vi "p49_1_trinterp.vi"() -> ()   [LabVIEW 2013]
uses:
  <vilib>/robotics/Kinematics/NI_Kinematics.lvlib
panel:
  out "Cartesian Motion 2":refnum<vi>(3d-picture)
  out "size(s) of P":i32[](array[numeric])
  out "Cartesian Motion":refnum<vi>(3d-picture)
  out "Cartesian Position":dbl[][](graph)
  out "RPY":dbl[][](graph)
  out "RPY":dbl[][](graph)
  out "Cartesian Position":dbl[][](graph)
  out "Ts(0)":picture
  out "size(s)":i32[](array[numeric])
  out "transformation matrix":picture
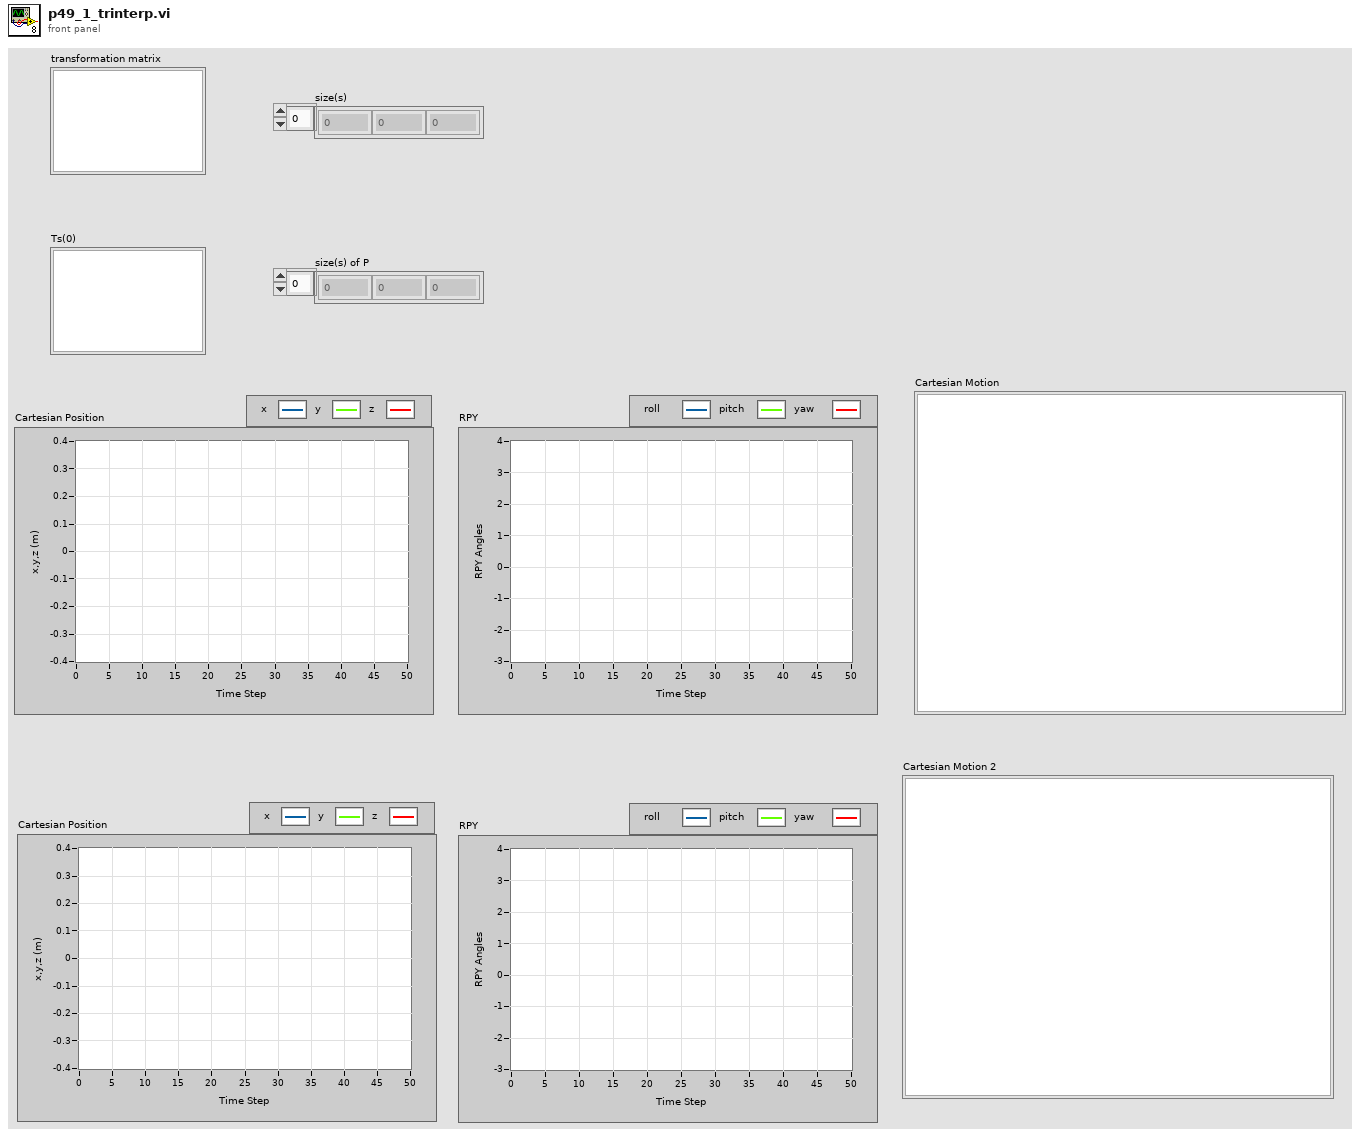
[diagram p1: front panel]
types:
  T1 = typedef "NI_Matrix.lvlib/RealMatrix.ctl" = dbl[][]
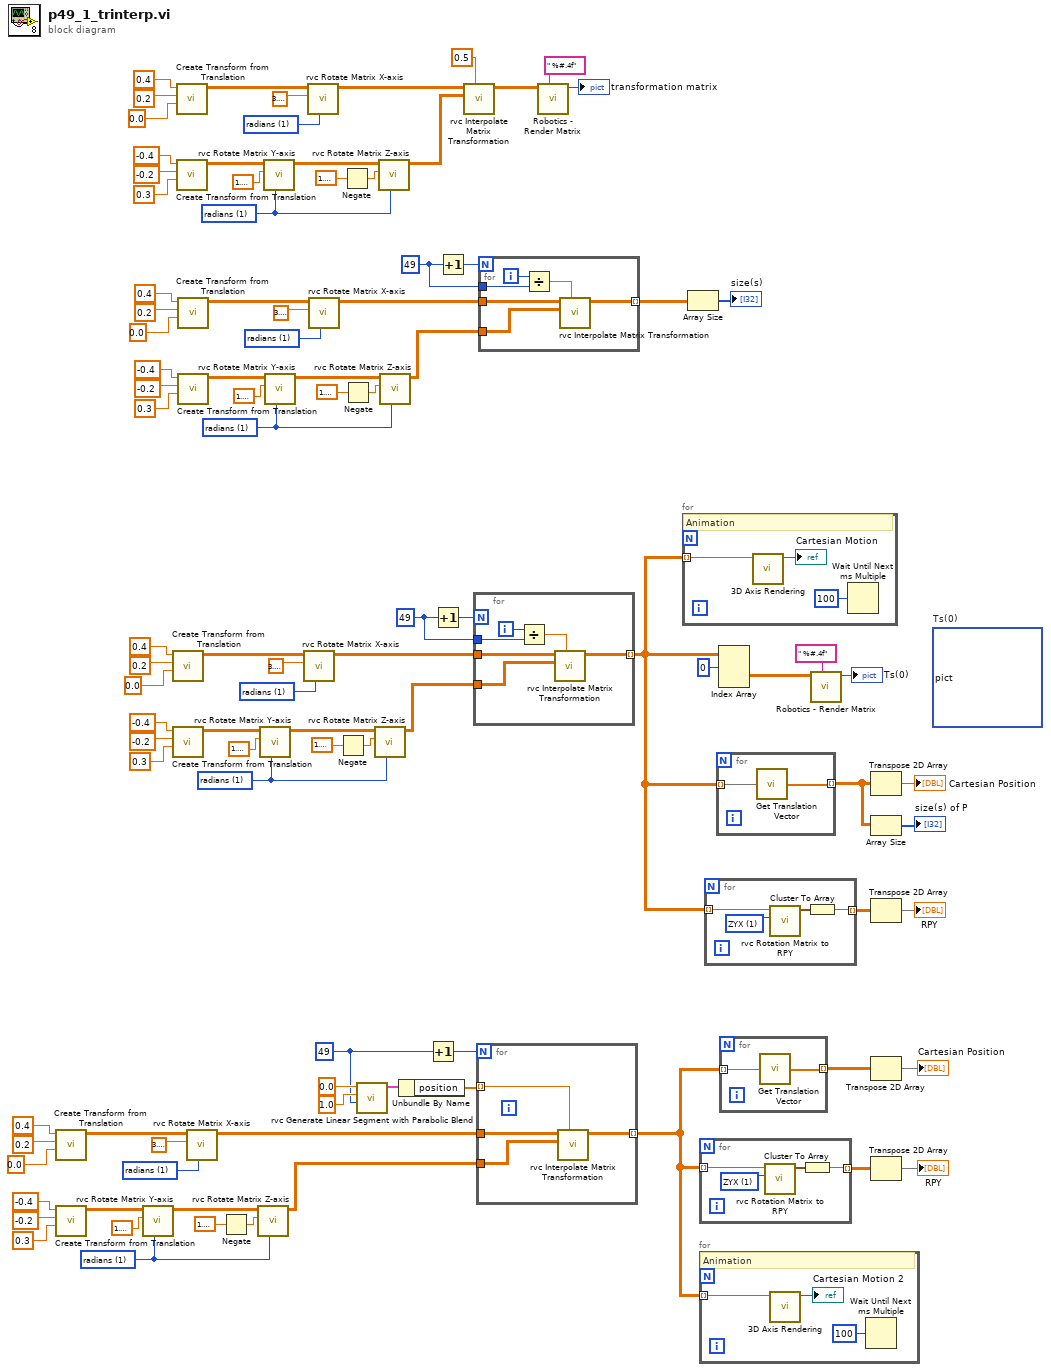
[diagram p0: block diagram]
diagram:
  (unwired) picture bytes[814]  # Ts(0)
  w26 = u16 1 items=["degree", "radians"] ("angle unit")
  w25 = u16 1 items=["degree", "radians"] ("angle unit")
  w7 = 49
  w41 = u16 1 items=["degree", "radians"] ("angle unit")
  w42 = u16 1 items=["degree", "radians"] ("angle unit")
  w39 = 49
  w80 = u16 1 items=["degree", "radians"] ("angle unit")
  w79 = u16 1 items=["degree", "radians"] ("angle unit")
  w82 = 49
  w85 = u16 1 items=["degree", "radians"] ("angle unit")
  w86 = u16 1 items=["degree", "radians"] ("angle unit")
  n1 = call <vilib>:"Create Transform from Translation.vi"("z"=0.0 ("Numeric"), "y"=0.2 ("Numeric"), "x"=0.4 ("Numeric")) -> ("transform"=w20:T1)  [unwired: 8 in]
  n2 = call <vilib>:"Create Transform from Translation.vi"("z"=0.3 ("Numeric"), "y"=-0.2 ("Numeric"), "x"=-0.4 ("Numeric")) -> ("transform"=w21:T1)  [unwired: 8 in]
  n3 = call "rvc Rotate Matrix Y-axis.vi"("angle unit"=w26, "angle"=1.5707963267948966, "rotation matrix in"=w21) -> ("rotation matrix"=w24:T1)  [unwired: 8 in]
  n4 = call <vilib>:"Create Transform from Translation.vi"("z"=0.0 ("Numeric"), "y"=0.2 ("Numeric"), "x"=0.4 ("Numeric")) -> ("transform"=w47:T1)  [unwired: 8 in]
  n5 = call <vilib>:"Create Transform from Translation.vi"("z"=0.3 ("Numeric"), "y"=-0.2 ("Numeric"), "x"=-0.4 ("Numeric")) -> ("transform"=w46:T1)  [unwired: 8 in]
  n6 = call <vilib>:"Create Transform from Translation.vi"("z"=0.0 ("Numeric"), "y"=0.2 ("Numeric"), "x"=0.4 ("Numeric")) -> ("transform"=w91:T1)  [unwired: 8 in]
  n7 = call <vilib>:"Create Transform from Translation.vi"("z"=0.3 ("Numeric"), "y"=-0.2 ("Numeric"), "x"=-0.4 ("Numeric")) -> ("transform"=w90:T1)  [unwired: 8 in]
  n8 = call <vilib>:"Create Transform from Translation.vi"("z"=0.0 ("Numeric"), "y"=0.2 ("Numeric"), "x"=0.4 ("Numeric")) -> ("transform"=w74:T1)  [unwired: 8 in]
  n9 = call <vilib>:"Create Transform from Translation.vi"("z"=0.3 ("Numeric"), "y"=-0.2 ("Numeric"), "x"=-0.4 ("Numeric")) -> ("transform"=w75:T1)  [unwired: 8 in]
  n10 = call "rvc Rotate Matrix X-axis.vi"("angle unit"=w25, "angle"=3.141592653589793, "rotation matrix in"=w20) -> ("rotation matrix"=w11:T1)  [unwired: 8 in]
  n11 = Negate(x=1.5707963267948966) -> (-x=w23:dbl)
  n12 = call "rvc Rotate Matrix Z-axis.vi"("angle unit"=w26, "angle"=w23, "rotation matrix in"=w24) -> ("rotation matrix"=w10:T1)  [unwired: 8 in]
  n13 = call "rvc Rotate Matrix Y-axis.vi"("angle unit"=w41, "angle"=1.5707963267948966, "rotation matrix in"=w46) -> ("rotation matrix"=w43:T1)  [unwired: 8 in]
  n14 = call "rvc Rotate Matrix Y-axis.vi"("angle unit"=w85, "angle"=1.5707963267948966, "rotation matrix in"=w90) -> ("rotation matrix"=w87:T1)  [unwired: 8 in]
  n15 = call "rvc Rotate Matrix Y-axis.vi"("angle unit"=w80, "angle"=1.5707963267948966, "rotation matrix in"=w75) -> ("rotation matrix"=w78:T1)  [unwired: 8 in]
  n16 = call "rvc Rotate Matrix X-axis.vi"("angle unit"=w42, "angle"=3.141592653589793, "rotation matrix in"=w47) -> ("rotation matrix"=w56:T1)  [unwired: 8 in]
  n17 = call "rvc Rotate Matrix X-axis.vi"("angle unit"=w86, "angle"=3.141592653589793, "rotation matrix in"=w91) -> ("rotation matrix"=w63:T1)  [unwired: 8 in]
  n18 = call "rvc Rotate Matrix X-axis.vi"("angle unit"=w79, "angle"=3.141592653589793, "rotation matrix in"=w74) -> ("rotation matrix"=w65:T1)  [unwired: 8 in]
  n19 = Negate(x=1.5707963267948966) -> (-x=w44:dbl)
  n20 = Negate(x=1.5707963267948966) -> (-x=w88:dbl)
  n21 = Negate(x=1.5707963267948966) -> (-x=w77:dbl)
  n22 = call "rvc Generate Linear Segment with Parabolic Blend.vi"("number of timesteps"=w7, "final position"=1.0, "initial position"=0.0) -> ("position"=w6:cluster{"time":dbl[], "position":dbl[]})  [unwired: 5 in, 3 out]
  n23 = call "rvc Rotate Matrix Z-axis.vi"("angle unit"=w41, "angle"=w44, "rotation matrix in"=w43) -> ("rotation matrix"=w57:T1)  [unwired: 8 in]
  n24 = call "rvc Rotate Matrix Z-axis.vi"("angle unit"=w85, "angle"=w88, "rotation matrix in"=w87) -> ("rotation matrix"=w62:T1)  [unwired: 8 in]
  n25 = call "rvc Rotate Matrix Z-axis.vi"("angle unit"=w80, "angle"=w77, "rotation matrix in"=w78) -> ("rotation matrix"=w64:T1)  [unwired: 8 in]
  n26 = Unbundle By Name(w6) -> ("position"=w5:dbl[])
  n27 = Increment(x=w7) -> (x+1=w27:i32)
  n28 = Increment(x=w39) -> (x+1=w40:i32)
  n29 = Increment(x=w82) -> (x+1=w81:i32)
  n30 = call "rvc Interpolate Matrix Transformation.vi"("ratio"=0.5, "final transformation"=w62, "initial transformation"=w63) -> ("interpolated matrix"=w60:T1)  [unwired: 8 in]
  n31 = for {
    N: w40 -> [_]
    tunnel: w56 -> [w102]
    tunnel: w57 -> [w103]
    tunnel: w39 -> [w104]
    tunnel: [w100] -> w4 mode=indexing
    i -> [w105]
    n32 = Divide(x=w105, y=w104) -> (x/y=w101:dbl)
    n33 = call "rvc Interpolate Matrix Transformation.vi"("ratio"=w101, "final transformation"=w103, "initial transformation"=w102) -> ("interpolated matrix"=w100:T1)  [unwired: 8 in]
  }
  n34 = for {
    N: w27 -> [_]
    tunnel: w11 -> [w108]
    tunnel: w10 -> [w109]
    tunnel: [w107] -> w1 mode=indexing
    tunnel: w5 -> [w106] mode=indexing
    # "Animation"
    n35 = call "rvc Interpolate Matrix Transformation.vi"("ratio"=w106, "final transformation"=w109, "initial transformation"=w108) -> ("interpolated matrix"=w107:T1)  [unwired: 8 in]
  }
  n36 = for {
    N: w81 -> [_]
    tunnel: w65 -> [w112]
    tunnel: w64 -> [w113]
    tunnel: w82 -> [w114]
    tunnel: [w110] -> w59 mode=indexing
    i -> [w115]
    n37 = Divide(x=w115, y=w114) -> (x/y=w111:dbl)
    n38 = call "rvc Interpolate Matrix Transformation.vi"("ratio"=w111, "final transformation"=w113, "initial transformation"=w112) -> ("interpolated matrix"=w110:T1)  [unwired: 8 in]
  }
  n39 = call "Robotics - Render Matrix.vi"("format string"=" %#.4f", "A"=w60) -> ("picture out"=→"transformation matrix":picture)  [unwired: 9 in]
  n40 = for {
    tunnel: w4 -> [w117] mode=indexing
    # "Animation"
    n41 = call "3D Axis Rendering.vi"("rotation matrix"=w117) -> ("SceneNode out"=→"Cartesian Motion":refnum<vi>)  [unwired: 10 in]
    n42 = Wait Until Next ms Multiple(millisecond multiple=u32 100) -> ()  [unwired: 1 out]
  }
  n43 = Array Size(array=w59) -> (size(s)=→"size(s)":i32[])
  n44 = for {
    tunnel: w1 -> [w122] mode=indexing
    tunnel: [w120] -> w30 mode=indexing
    w119 = u16 1 items=["XYZ", "ZYX"] ("Convension")
    n45 = call "rvc Rotation Matrix to RPY.vi"("Convension"=w119, "rotation matrix"=w122) -> ("angles"=w121:cluster{"roll":dbl, "pitch":dbl, "yaw":dbl})  [unwired: 9 in]
    n46 = Cluster To Array(cluster=w121) -> (array=w120:dbl[])
  }
  n47 = for {
    tunnel: w1 -> [w124] mode=indexing
    # "Animation"
    n48 = call "3D Axis Rendering.vi"("rotation matrix"=w124) -> ("SceneNode out"=→"Cartesian Motion 2":refnum<vi>)  [unwired: 10 in]
    n49 = Wait Until Next ms Multiple(millisecond multiple=u32 100) -> ()  [unwired: 1 out]
  }
  n50 = for {
    tunnel: w4 -> [w129] mode=indexing
    tunnel: [w127] -> w33 mode=indexing
    w126 = u16 1 items=["XYZ", "ZYX"] ("Convension")
    n51 = call "rvc Rotation Matrix to RPY.vi"("Convension"=w126, "rotation matrix"=w129) -> ("angles"=w128:cluster{"roll":dbl, "pitch":dbl, "yaw":dbl})  [unwired: 9 in]
    n52 = Cluster To Array(cluster=w128) -> (array=w127:dbl[])
  }
  n53 = for {
    tunnel: w4 -> [w131] mode=indexing
    tunnel: [w130] -> w2 mode=indexing
    n54 = call <vilib>:"Get Translation Vector.vi"("transform"=w131) -> ("translation vector"=w130:dbl[])
  }
  n55 = Index Array(array=w4, index (dim 0)=0 ("index (page)")) -> (element=w35:dbl[][])  [unwired: 2 in]
  n56 = for {
    tunnel: w1 -> [w133] mode=indexing
    tunnel: [w132] -> w28 mode=indexing
    n57 = call <vilib>:"Get Translation Vector.vi"("transform"=w133) -> ("translation vector"=w132:dbl[])
  }
  n58 = call "Robotics - Render Matrix.vi"("format string"=" %#.4f", "A"=w35) -> ("picture out"=→"Ts(0)":picture)  [unwired: 9 in]
  n59 = Transpose 2D Array(2D array=w2) -> (transposed array=→"Cartesian Position":dbl[][])
  n60 = Array Size(array=w2) -> (size(s)=→"size(s) of P":i32[])
  n61 = Transpose 2D Array(2D array=w33) -> (transposed array=→"RPY":dbl[][])
  n62 = Transpose 2D Array(2D array=w28) -> (transposed array=→"Cartesian Position":dbl[][])
  n63 = Transpose 2D Array(2D array=w30) -> (transposed array=→"RPY":dbl[][])
